vi "main.vi"() -> ()   [LabVIEW 2019]
panel:
  in  "udl":bool
  in  "rock":bool
  in  "unrock":bool
  in  "index":bool
  in  "停止":bool
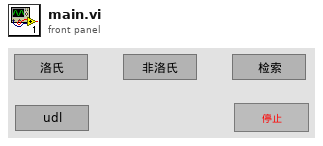
[diagram p1: front panel]
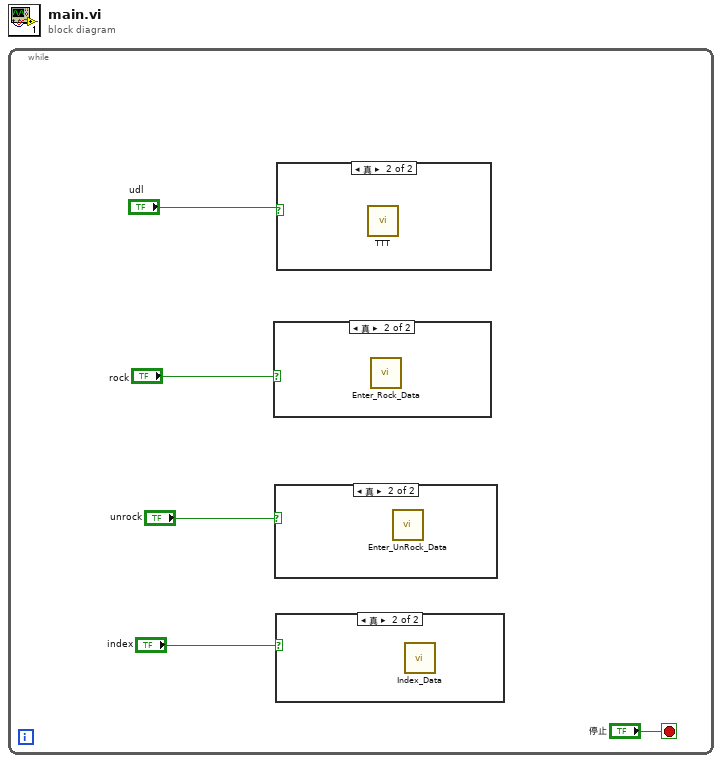
[diagram p0: block diagram]
diagram:
  n1 = while {
    stop <- "停止" stop-if-true
    n2 = case shown="真" "rock" {
      frame False {
      }
      frame True {
        n3 = call "Enter_Rock_Data.vi"() -> ()  [unwired: 12 in]
      }
    }
    n4 = case shown="真" "unrock" {
      frame False {
      }
      frame True {
        n5 = call "Enter_UnRock_Data.vi"() -> ()  [unwired: 12 in]
      }
    }
    n6 = case shown="真" "index" {
      frame False {
      }
      frame True {
        n7 = call "Index_Data.vi"() -> ()  [unwired: 12 in]
      }
    }
    n8 = case shown="真" "udl" {
      frame False {
      }
      frame True {
        n9 = call "TTT.vi"() -> ()  [unwired: 12 in]
      }
    }
  }
